vi "Camera_Config_Global_Attributes_2.0.vi"(7 "Camera":T5, 8 "error in (no error)":errorcluster, 10 "Refnum in":T2, 11 "Data":T1={"Camera 1"={"Camera1"="", "Cam 1"=FALSE, "CAM1 Model"=enum."a2A5328-15ucBAS", "Cam1 ID"=0}, "Camera 2"={"Camera2"="", "Cam 2"=FALSE, "CAM2 Model"=enum."a2A5328-15ucBAS", "Cam2 ID"=0}, "Image"={"Camera1_Img"=refnum, "Camera2_Img"=refnum, "Img1_Orig_Disp"=refnum, "Img2_Orig_Disp"=refnum, "Img1_Orig_RGB"=refnum, "Img2_Orig_RGB"=refnum, "Blue_Plane_Extract"=refnum, "Subtracted_Plane"=refnum, "Img1_Binary"=refnum, "Img2_Binary"=refnum, "Crop_Mask"=refnum, "Img1_Save"=refnum, "Img2_Save"=refnum, "Img1_Cali_Full"=refnum, "Img2_Cali_Full"=refnum, "Img1_Cali_Detect"=refnum, "Img2_Cali_Detect"=refnum}, "Ques"={"Cam 1 queue"=refnum, "Cam 2 queue"=refnum, "Cam 1 - save queue"=refnum, "Cam 2 - save queue"=refnum, "Image Process Queue Size"=500, "Image Save Queue Size"=500, "Overload threshold"=500, "Max large object threshold"=0}, "Arduino SRS"={"Pinch-valve"="", "Actuator"=FALSE, "Open(T)/Close(F)"=FALSE, "Arduino Uno"=""}, "Pump"={"Port"="", "Connection"=FALSE, "Flush Size"=0, "Command"="", "Pump Size"=enum."None", "Pump"=""}, "Camera settings"={"Detection settings"={"Sample size threshold"=500, "Detection Region %"=30.0, "Timeout Sample"=200}, "Lens/camera settings"={"Aperture"=enum."Item 0", "Legacy Cam Attributes"=FALSE, "Max Framerate"=100, "Exposure Time"=1000.0, "Framerate"=15}, "Crop settings"={"Cam1"={"Rectangle 1"={"Left"=0, "Top"=0, "Right"=0, "Bottom"=0, "Rotation"=0.0}, "Camera Orientation 1"="", "Pixel to mm 1"=0.0}, "Cam2"={"Rectangle 2"={"Left"=0, "Top"=0, "Right"=0, "Bottom"=0, "Rotation"=0.0}, "Camera Orientation 2"="", "Pixel to mm 2"=0.0}}}, "Arduino ISS"={"Mega F3"="", "Phase3"=FALSE, "Barcode"="", "Sorting sys."=FALSE, "Initial size"=0.0, "Size Interval"=0.0, "Mun. of containers"=0.0, "Container nr."=0.0, "Arduino Mega"=""}, "Img_Capt"=FALSE, "Empty_Refill"=FALSE, "I don't think is in use"={"Light intensity"=100}, "Extended setup"={"Location"="Station", "Latitude"="Station", "Longitude"="Station", "Determiner"="Station", "Sex"="Station", "Station"="", "Collection date"=""}, "Main interface"={"Sample Name"="Test Sample", "Operator"="JFR", "Species Name"="", "Other Notes"=""}, "Tap1"=0, "SystemVersion"=0, "System Serial"="", "Exit"=FALSE, "Kuvette Full"=FALSE, "Core JKI"={"Current VI Reference"=refnum, "Close Panel on Exit?"=FALSE}, "Calibration"={"Calibration 1"=path "C:/Users/au540322/Desktop/IHS_Project/images/Debris/Debris_0/Debris_0_2019_06_01-23-32-49-686.PNG", "Calibration 2"=path "C:/Users/au540322/Desktop/IHS_Project/images/Debris/Debris_0/Debris_0_2019_06_01-23-32-49-686.PNG", "Detect 1"=path "C:/Users/au540322/Desktop/IHS_Project/images/Debris/Debris_0/Debris_0_2019_06_01-23-32-49-686.PNG", "Detect 2"=path "C:/Users/au540322/Desktop/IHS_Project/images/Debris/Debris_0/Debris_0_2019_06_01-23-32-49-686.PNG"}, "Flush Insect"=FALSE, "Auto Flush"=FALSE} {"SystemVersion" items=["Standard", "XL"]; "Tap1" items=["Session Data", "Extended Setup", "Buffer", "Camera", "Dispenser", "Stats", "Connections"]; "I don't think is in use"."Light intensity" scale=0.0..100.0; "Camera settings"."Crop settings"."Cam2"."Rectangle 2"."Rotation" format="%.2f"; "Camera settings"."Crop settings"."Cam2"."Rectangle 2"."Left" scale=0.0..1024.0; "Camera settings"."Crop settings"."Cam2"."Rectangle 2"."Right" scale=0.0..1024.0; "Camera settings"."Crop settings"."Cam1"."Rectangle 1"."Rotation" format="%.2f"; "Camera settings"."Crop settings"."Cam1"."Rectangle 1"."Left" scale=0.0..1024.0; "Camera settings"."Crop settings"."Cam1"."Rectangle 1"."Right" scale=0.0..1024.0; "Camera settings"."Lens/camera settings"."Framerate" min=1; "Camera settings"."Lens/camera settings"."Max Framerate" min=1; "Camera settings"."Detection settings"."Sample size threshold" min=1; "Pump"."Flush Size" min=0 max=6000 step=100; "Ques"."Overload threshold" min=1; "Ques"."Image Save Queue Size" min=1; "Ques"."Image Process Queue Size" min=1}) -> (0 "error out":errorcluster, 2 "Refnum out":T2, 3 "Data Out":T1={"Camera 1"={"Camera1"="", "Cam 1"=FALSE, "CAM1 Model"=enum."a2A5328-15ucBAS", "Cam1 ID"=0}, "Camera 2"={"Camera2"="", "Cam 2"=FALSE, "CAM2 Model"=enum."a2A5328-15ucBAS", "Cam2 ID"=0}, "Image"={"Camera1_Img"=refnum, "Camera2_Img"=refnum, "Img1_Orig_Disp"=refnum, "Img2_Orig_Disp"=refnum, "Img1_Orig_RGB"=refnum, "Img2_Orig_RGB"=refnum, "Blue_Plane_Extract"=refnum, "Subtracted_Plane"=refnum, "Img1_Binary"=refnum, "Img2_Binary"=refnum, "Crop_Mask"=refnum, "Img1_Save"=refnum, "Img2_Save"=refnum, "Img1_Cali_Full"=refnum, "Img2_Cali_Full"=refnum, "Img1_Cali_Detect"=refnum, "Img2_Cali_Detect"=refnum}, "Ques"={"Cam 1 queue"=refnum, "Cam 2 queue"=refnum, "Cam 1 - save queue"=refnum, "Cam 2 - save queue"=refnum, "Image Process Queue Size"=500, "Image Save Queue Size"=500, "Overload threshold"=500, "Max large object threshold"=0}, "Arduino SRS"={"Pinch-valve"="", "Actuator"=FALSE, "Open(T)/Close(F)"=FALSE, "Arduino Uno"=""}, "Pump"={"Port"="", "Connection"=FALSE, "Flush Size"=0, "Command"="", "Pump Size"=enum."None", "Pump"=""}, "Camera settings"={"Detection settings"={"Sample size threshold"=500, "Detection Region %"=30.0, "Timeout Sample"=200}, "Lens/camera settings"={"Aperture"=enum."Item 0", "Legacy Cam Attributes"=FALSE, "Max Framerate"=100, "Exposure Time"=1000.0, "Framerate"=15}, "Crop settings"={"Cam1"={"Rectangle 1"={"Left"=0, "Top"=0, "Right"=0, "Bottom"=0, "Rotation"=0.0}, "Camera Orientation 1"="", "Pixel to mm 1"=0.0}, "Cam2"={"Rectangle 2"={"Left"=0, "Top"=0, "Right"=0, "Bottom"=0, "Rotation"=0.0}, "Camera Orientation 2"="", "Pixel to mm 2"=0.0}}}, "Arduino ISS"={"Mega F3"="", "Phase3"=FALSE, "Barcode"="", "Sorting sys."=FALSE, "Initial size"=0.0, "Size Interval"=0.0, "Mun. of containers"=0.0, "Container nr."=0.0, "Arduino Mega"=""}, "Img_Capt"=FALSE, "Empty_Refill"=FALSE, "I don't think is in use"={"Light intensity"=100}, "Extended setup"={"Location"="Station", "Latitude"="Station", "Longitude"="Station", "Determiner"="Station", "Sex"="Station", "Station"="", "Collection date"=""}, "Main interface"={"Sample Name"="Test Sample", "Operator"="JFR", "Species Name"="", "Other Notes"=""}, "Tap1"=0, "SystemVersion"=0, "System Serial"="", "Exit"=FALSE, "Kuvette Full"=FALSE, "Core JKI"={"Current VI Reference"=refnum, "Close Panel on Exit?"=FALSE}, "Calibration"={"Calibration 1"=path "C:/Users/au540322/Desktop/IHS_Project/images/Debris/Debris_0/Debris_0_2019_06_01-23-32-49-686.PNG", "Calibration 2"=path "C:/Users/au540322/Desktop/IHS_Project/images/Debris/Debris_0/Debris_0_2019_06_01-23-32-49-686.PNG", "Detect 1"=path "C:/Users/au540322/Desktop/IHS_Project/images/Debris/Debris_0/Debris_0_2019_06_01-23-32-49-686.PNG", "Detect 2"=path "C:/Users/au540322/Desktop/IHS_Project/images/Debris/Debris_0/Debris_0_2019_06_01-23-32-49-686.PNG"}, "Flush Insect"=FALSE, "Auto Flush"=FALSE} {"SystemVersion" items=["Standard", "XL"]; "Tap1" items=["Session Data", "Extended Setup", "Buffer", "Camera", "Dispenser", "Stats", "Connections"]; "I don't think is in use"."Light intensity" scale=0.0..100.0; "Camera settings"."Crop settings"."Cam2"."Rectangle 2"."Rotation" format="%.2f"; "Camera settings"."Crop settings"."Cam2"."Rectangle 2"."Left" scale=0.0..1024.0; "Camera settings"."Crop settings"."Cam2"."Rectangle 2"."Right" scale=0.0..1024.0; "Camera settings"."Crop settings"."Cam1"."Rectangle 1"."Rotation" format="%.2f"; "Camera settings"."Crop settings"."Cam1"."Rectangle 1"."Left" scale=0.0..1024.0; "Camera settings"."Crop settings"."Cam1"."Rectangle 1"."Right" scale=0.0..1024.0; "Camera settings"."Lens/camera settings"."Framerate" min=1; "Camera settings"."Lens/camera settings"."Max Framerate" min=1; "Camera settings"."Detection settings"."Sample size threshold" min=1; "Pump"."Flush Size" min=0 max=6000 step=100; "Ques"."Overload threshold" min=1; "Ques"."Image Save Queue Size" min=1; "Ques"."Image Process Queue Size" min=1})   [LabVIEW 2024]
uses:
  <vilib>/userDefined/High Color/IMAQdx.ctl
  Camera_ID.ctl
  controls/Data_JKI.ctl
  <vilib>/vision/Image Controls.llb/IMAQ Image.ctl
  <resource>/objmgr/imaqdx.rc
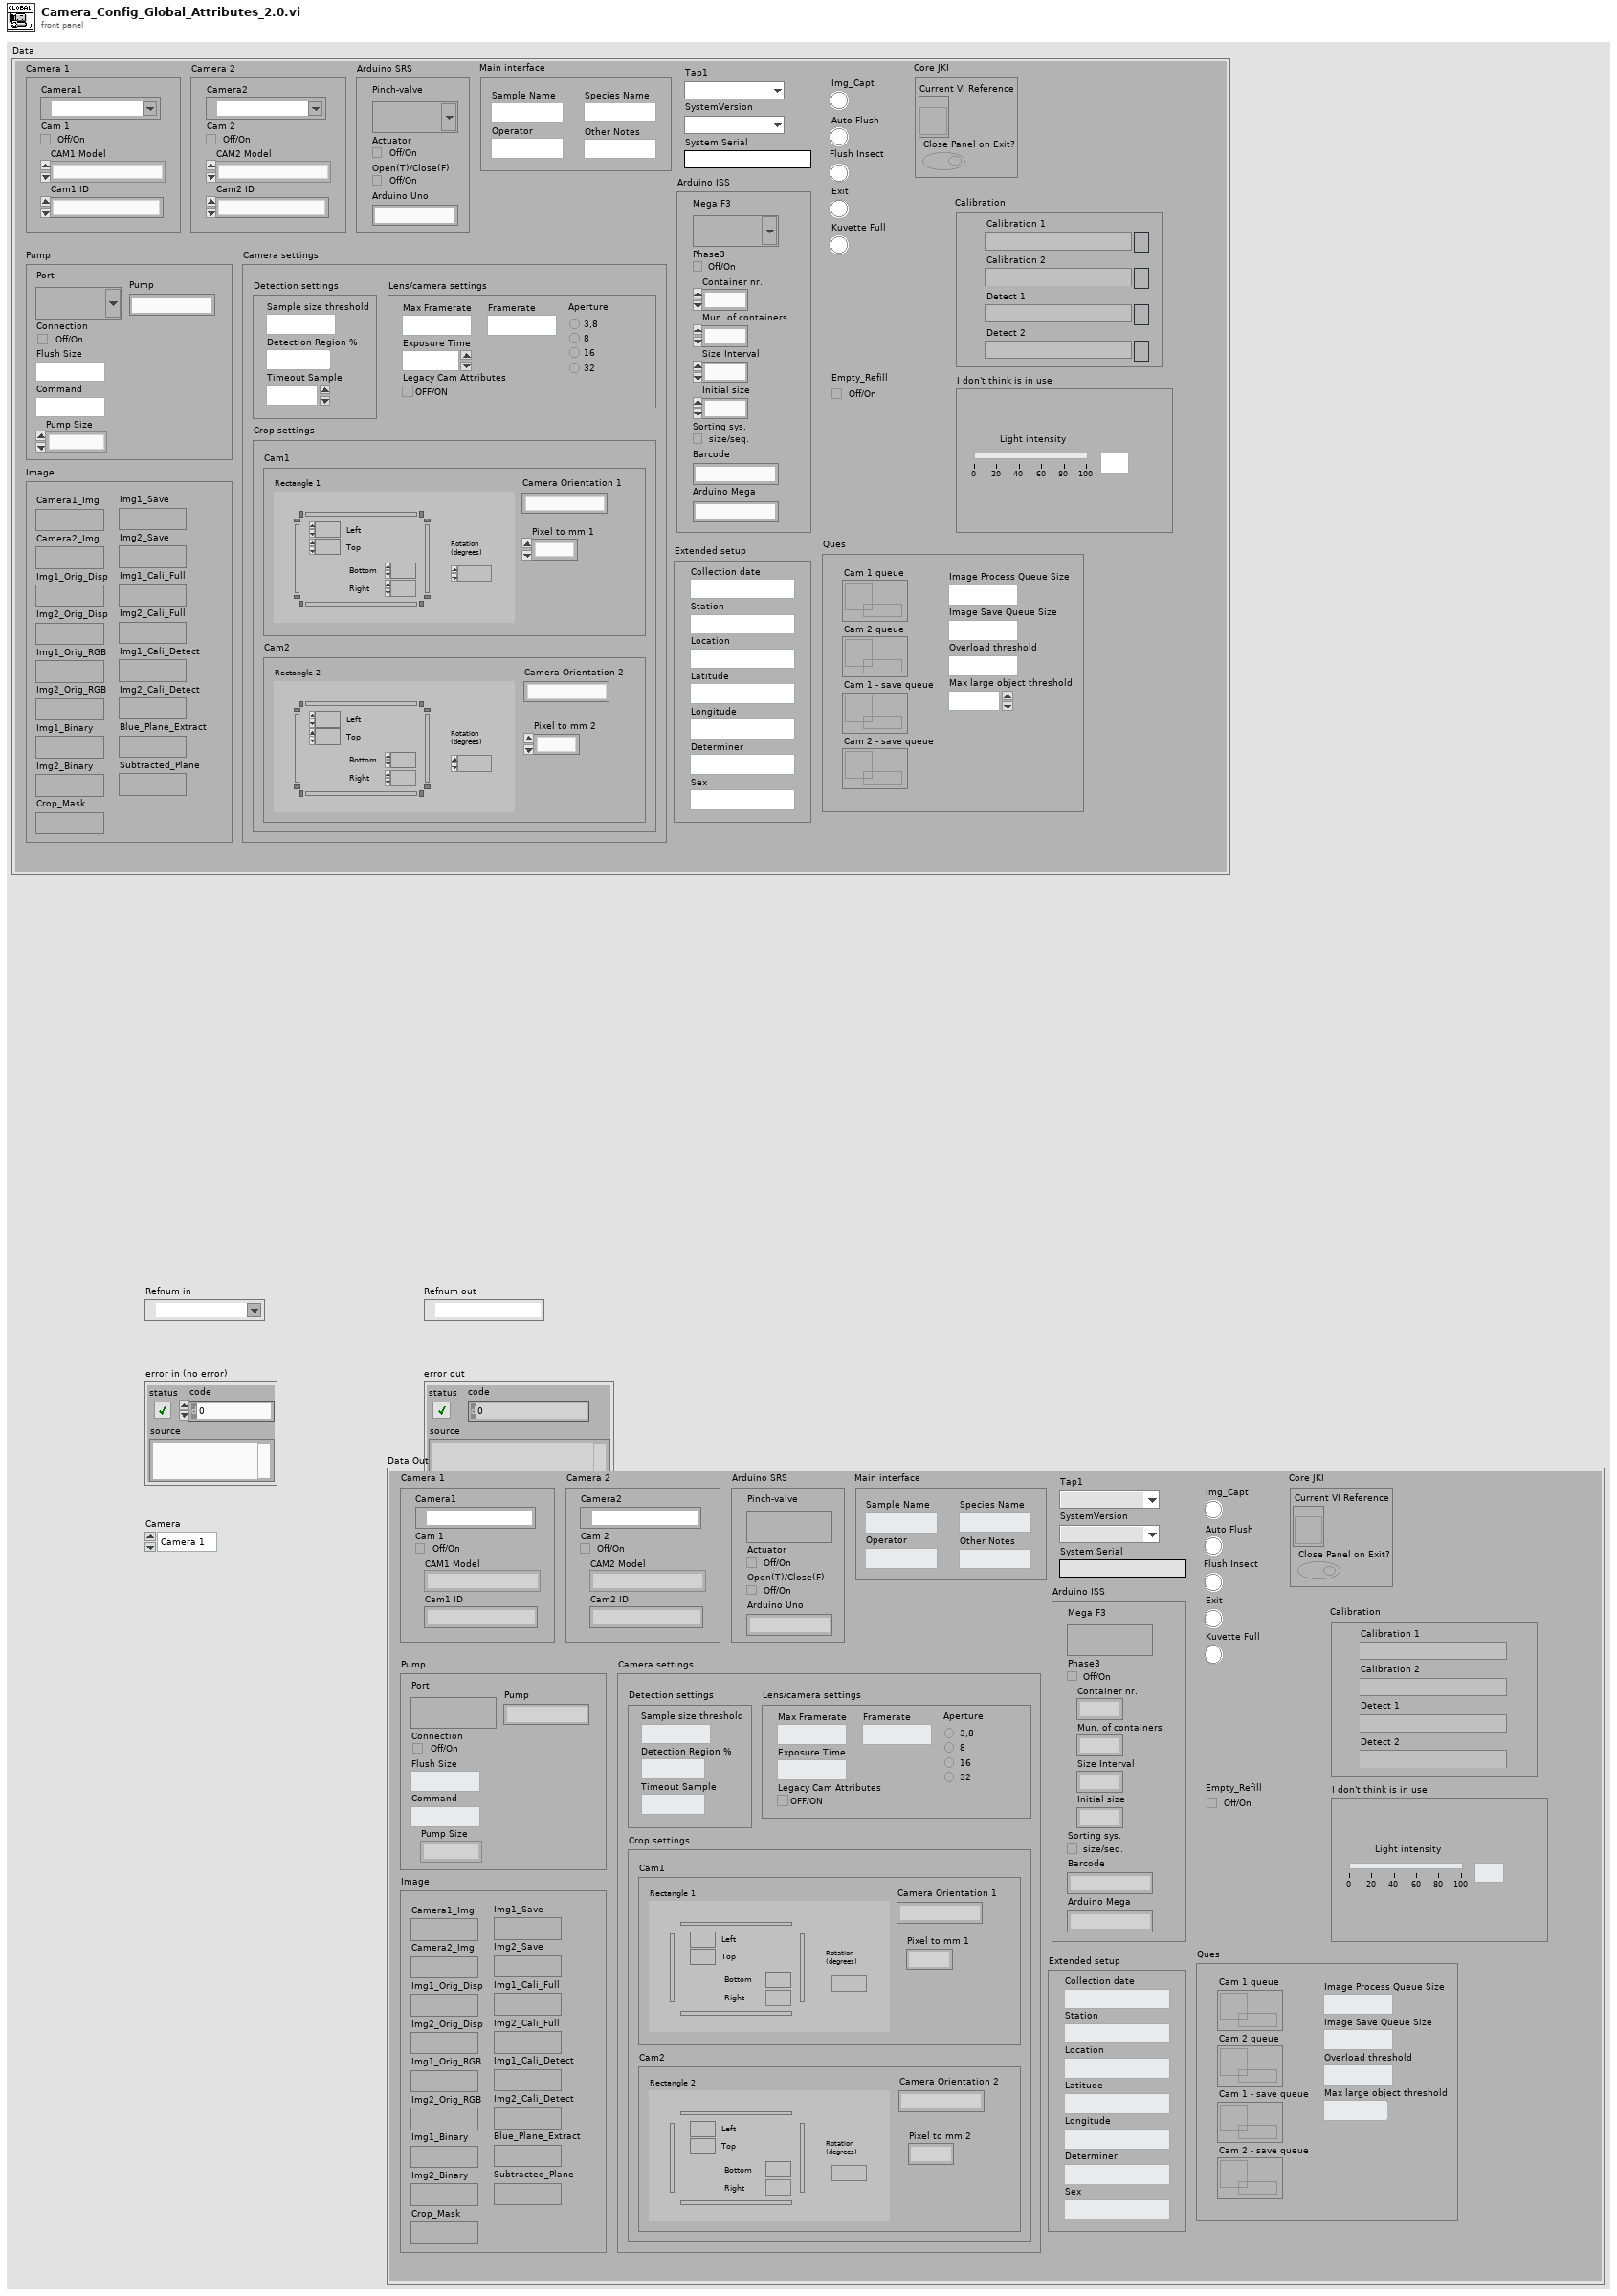
[diagram p1: front panel]
types:
  T1 = typedef "Data_JKI.ctl" = cluster{"Camera 1":cluster{"Camera1":T2, "Cam 1":bool, "CAM1 Model":enum16{"a2A5328-15ucBAS", "acA1920-155uc"}, "Cam1 ID":i32}, "Camera 2":cluster{"Camera2":T2, "Cam 2":bool, "CAM2 Model":enum16{"a2A5328-15ucBAS", "acA1920-155uc"}, "Cam2 ID":i32}, "Image":cluster{"Camera1_Img":T3, "Camera2_Img":T3, "Img1_Orig_Disp":T3, "Img2_Orig_Disp":T3, "Img1_Orig_RGB":T3, "Img2_Orig_RGB":T3, "Blue_Plane_Extract":T3, "Subtracted_Plane":T3, "Img1_Binary":T3, "Img2_Binary":T3, "Crop_Mask":T3, "Img1_Save":T3, "Img2_Save":T3, "Img1_Cali_Full":T3, "Img2_Cali_Full":T3, "Img1_Cali_Detect":T3, "Img2_Cali_Detect":T3}, "Ques":cluster{"Cam 1 queue":refnum<queue>, "Cam 2 queue":refnum<queue>, "Cam 1 - save queue":refnum<queue>, "Cam 2 - save queue":refnum<queue>, "Image Process Queue Size":i32, "Image Save Queue Size":i32, "Overload threshold":i32, "Max large object threshold":i32}, "Arduino SRS":cluster{"Pinch-valve":refnum<visa-resource-name>, "Actuator":bool, "Open(T)/Close(F)":bool, "Arduino Uno":string}, "Pump":cluster{"Port":refnum<visa-resource-name>, "Connection":bool, "Flush Size":i32, "Command":string, "Pump Size":enum16{"None", "Small", "Large"}, "Pump":string}, "Camera settings":cluster{"Detection settings":cluster{"Sample size threshold":i32, "Detection Region %":dbl, "Timeout Sample":i32}, "Lens/camera settings":cluster{"Aperture":enum32{"Item 0", "Item 1", "Item 2", "Item 3"}, "Legacy Cam Attributes":bool, "Max Framerate":i32, "Exposure Time":dbl, "Framerate":i32}, "Crop settings":cluster{"Cam1":cluster{"Rectangle 1":T4, "Camera Orientation 1":string, "Pixel to mm 1":dbl}, "Cam2":cluster{"Rectangle 2":T4, "Camera Orientation 2":string, "Pixel to mm 2":dbl}}}, "Arduino ISS":cluster{"Mega F3":refnum<visa-resource-name>, "Phase3":bool, "Barcode":string, "Sorting sys.":bool, "Initial size":dbl, "Size Interval":dbl, "Mun. of containers":dbl, "Container nr.":dbl, "Arduino Mega":string}, "Img_Capt":bool, "Empty_Refill":bool, "I don't think is in use":cluster{"Light intensity":i32}, "Extended setup":cluster{"Location":string, "Latitude":string, "Longitude":string, "Determiner":string, "Sex":string, "Station":string, "Collection date":string}, "Main interface":cluster{"Sample Name":string, "Operator":string, "Species Name":string, "Other Notes":string}, "Tap1":u16, "SystemVersion":u16, "System Serial":string, "Exit":bool, "Kuvette Full":bool, "Core JKI":cluster{"Current VI Reference":refnum<vi>, "Close Panel on Exit?":bool}, "Calibration":cluster{"Calibration 1":path, "Calibration 2":path, "Detect 1":path, "Detect 2":path}, "Flush Insect":bool, "Auto Flush":bool}
  T2 = typedef "IMAQdx.ctl" = refnum<k21>
  T3 = typedef "IMAQ Image.ctl" = refnum<image>
  T4 = typedef "IMAQ Rectangle" = cluster{"Left":i32, "Top":i32, "Right":i32, "Bottom":i32, "Rotation":dbl}
  T5 = typedef "Camera_ID.ctl" = enum16{"Camera 1", "Camera 2"}
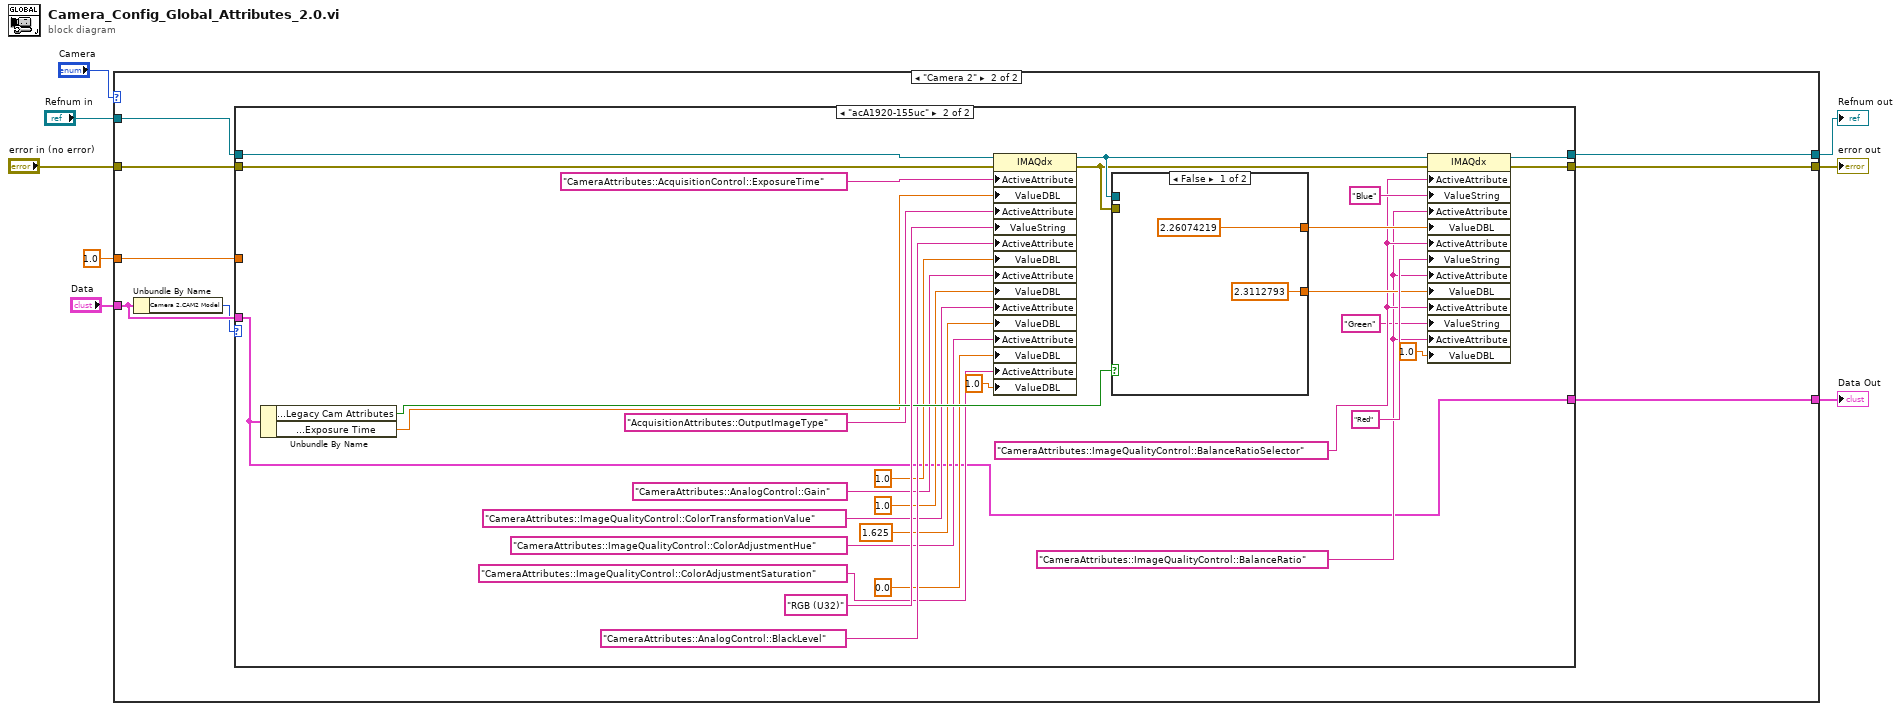
[diagram p0: block diagram]
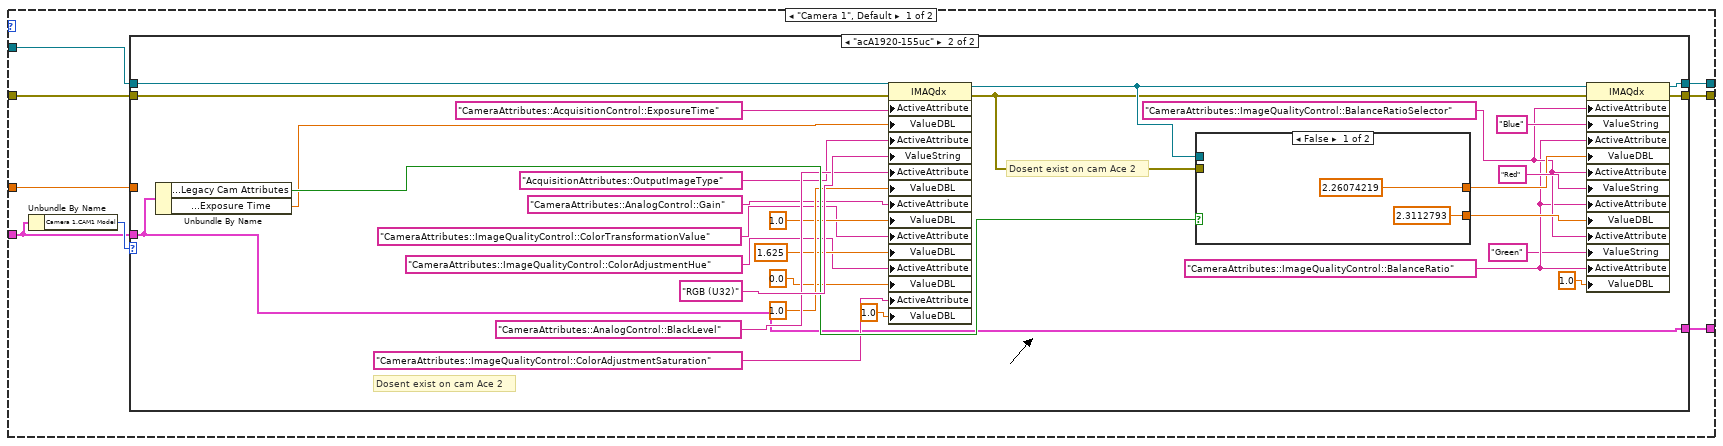
[diagram p2: hidden frame]
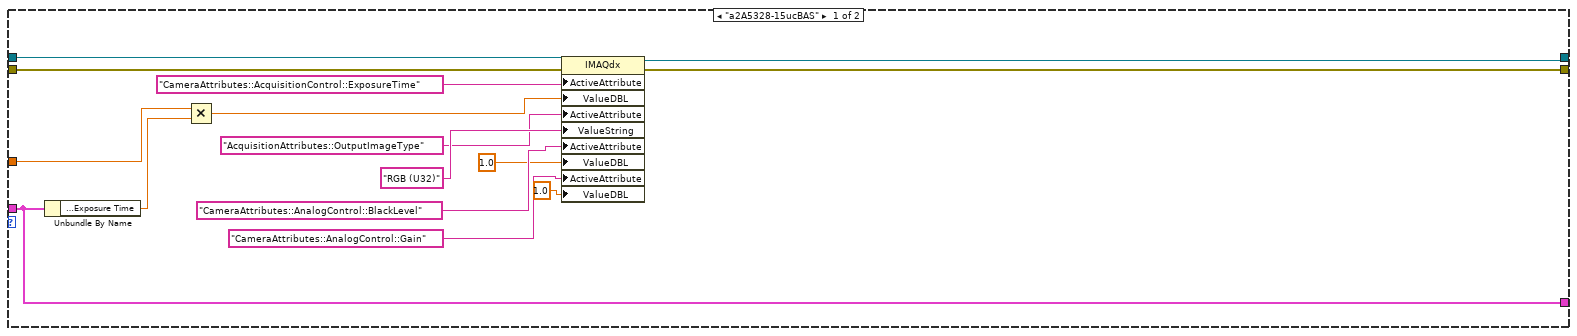
[diagram p3: hidden frame]
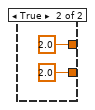
[diagram p4: hidden frame]
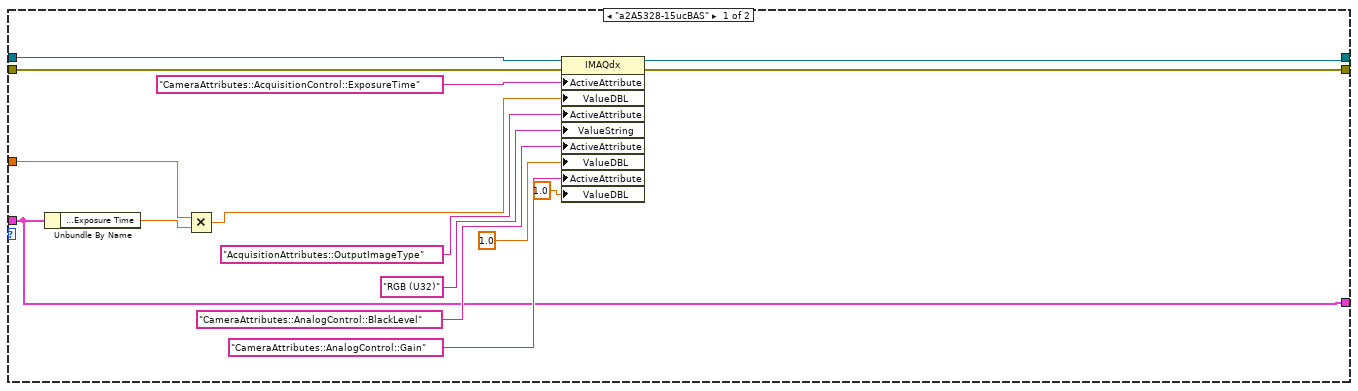
[diagram p5: hidden frame]
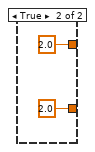
[diagram p6: hidden frame]
diagram:
  n1 = case shown="\"Camera 2\"" "Camera" {
    tunnel: "Data" -> [w13 w73]
    tunnel: "error in (no error)" -> [w14 w72]
    tunnel: [w15 w71] -> w7
    tunnel: "Refnum in" -> [w10 w69]
    tunnel: [w12 w68] -> w4
    tunnel: [w11 w67] -> w3
    tunnel: 1.0 ("x") -> [w9 w66]
    frame "Camera 1", Default {
      n2 = Unbundle By Name(w13) -> ("Camera 1.CAM1 Model"=w16:enum16{"a2A5328-15ucBAS", "acA1920-155uc"})
      n3 = case shown="\"acA1920-155uc\"" w16 {
        tunnel: w13 -> [w27 w34]
        tunnel: w14 -> [w31 w37]
        tunnel: [w29 w36] -> w15
        tunnel: [w27 w34] -> w12
        tunnel: [w28 w35] -> w11
        tunnel: w10 -> [w30 w33]
        tunnel: w9 -> [w19 _]
        frame "a2A5328-15ucBAS" {
          n4 = Unbundle By Name(w27) -> ("Camera settings.Lens/camera settings.Exposure Time"=w18:dbl)
          n5 = Multiply(x=w19, y=w18) -> (x*y=w17:dbl)
          n6 = property class="IMAQdx"(reference=w30, error in=w31, "ActiveAttribute"="CameraAttributes::AcquisitionControl::ExposureTime", "ValueDBL"=w17, "ActiveAttribute"="AcquisitionAttributes::OutputImageType", "ValueString"="RGB (U32)", "ActiveAttribute"="CameraAttributes::AnalogControl::BlackLevel", "ValueDBL"=1.0, "ActiveAttribute"="CameraAttributes::AnalogControl::Gain", "ValueDBL"=1.0) -> (reference out=w28:T2, error out=w29:errorcluster)
        }
        frame "acA1920-155uc" {
          w42 = "CameraAttributes::ImageQualityControl::BalanceRatio" ("ActiveAttribute")
          w43 = "CameraAttributes::ImageQualityControl::BalanceRatioSelector" ("ActiveAttribute")
          # "Dosent exist on cam Ace 2"
          # "Dosent exist on cam Ace 2"
          n7 = Unbundle By Name(w34) -> ("Camera settings.Lens/camera settings.Legacy Cam Attributes"=w58:bool, "Camera settings.Lens/camera settings.Exposure Time"=w32:dbl)
          n8 = property class="IMAQdx"(reference=w33, error in=w37, "ActiveAttribute"="CameraAttributes::AcquisitionControl::ExposureTime", "ValueDBL"=w32, "ActiveAttribute"="AcquisitionAttributes::OutputImageType", "ValueString"="RGB (U32)", "ActiveAttribute"="CameraAttributes::AnalogControl::BlackLevel", "ValueDBL"=1.0, "ActiveAttribute"="CameraAttributes::AnalogControl::Gain", "ValueDBL"=1.0, "ActiveAttribute"="CameraAttributes::ImageQualityControl::ColorTransformationValue", "ValueDBL"=1.625, "ActiveAttribute"="CameraAttributes::ImageQualityControl::ColorAdjustmentHue", "ValueDBL"=0.0, "ActiveAttribute"="CameraAttributes::ImageQualityControl::ColorAdjustmentSaturation", "ValueDBL"=1.0) -> (reference out=w60:T2, error out=w59:errorcluster)
          n9 = case shown="False" w58 {
            tunnel: w60 -> [_ _]
            tunnel: w59 -> [_ _]
            tunnel: [2.26074219 ("ValueDBL") 2.0 ("ValueDBL")] -> w55
            tunnel: [2.3112793 ("ValueDBL") 2.0 ("ValueDBL")] -> w54
            frame False {
            }
            frame True {
            }
          }
          n10 = property class="IMAQdx"(reference=w60, error in=w59, "ActiveAttribute"=w43, "ValueString"="Blue", "ActiveAttribute"=w42, "ValueDBL"=w55, "ActiveAttribute"=w43, "ValueString"="Red", "ActiveAttribute"=w42, "ValueDBL"=w54, "ActiveAttribute"=w43, "ValueString"="Green", "ActiveAttribute"=w42, "ValueDBL"=1.0) -> (reference out=w35:T2, error out=w36:errorcluster)
        }
      }
    }
    frame "Camera 2" {
      n11 = Unbundle By Name(w73) -> ("Camera 2.CAM2 Model"=w70:enum16{"a2A5328-15ucBAS", "acA1920-155uc"})
      n12 = case shown="\"acA1920-155uc\"" w70 {
        tunnel: w73 -> [w79 w90]
        tunnel: w72 -> [w81 w94]
        tunnel: [w78 w93] -> w71
        tunnel: w69 -> [w80 w91]
        tunnel: [w79 w90] -> w68
        tunnel: [w77 w92] -> w67
        tunnel: w66 -> [w74 _]
        frame "a2A5328-15ucBAS" {
          n13 = Unbundle By Name(w79) -> ("Camera settings.Lens/camera settings.Exposure Time"=w76:dbl)
          n14 = Multiply(x=w74, y=w76) -> (x*y=w75:dbl)
          n15 = property class="IMAQdx"(reference=w80, error in=w81, "ActiveAttribute"="CameraAttributes::AcquisitionControl::ExposureTime", "ValueDBL"=w75, "ActiveAttribute"="AcquisitionAttributes::OutputImageType", "ValueString"="RGB (U32)", "ActiveAttribute"="CameraAttributes::AnalogControl::BlackLevel", "ValueDBL"=1.0, "ActiveAttribute"="CameraAttributes::AnalogControl::Gain", "ValueDBL"=1.0) -> (reference out=w77:T2, error out=w78:errorcluster)
        }
        frame "acA1920-155uc" {
          w99 = "CameraAttributes::ImageQualityControl::BalanceRatio" ("ActiveAttribute")
          w100 = "CameraAttributes::ImageQualityControl::BalanceRatioSelector" ("ActiveAttribute")
          n16 = Unbundle By Name(w90) -> ("Camera settings.Lens/camera settings.Legacy Cam Attributes"=w115:bool, "Camera settings.Lens/camera settings.Exposure Time"=w89:dbl)
          n17 = property class="IMAQdx"(reference=w91, error in=w94, "ActiveAttribute"="CameraAttributes::AcquisitionControl::ExposureTime", "ValueDBL"=w89, "ActiveAttribute"="AcquisitionAttributes::OutputImageType", "ValueString"="RGB (U32)", "ActiveAttribute"="CameraAttributes::AnalogControl::BlackLevel", "ValueDBL"=1.0, "ActiveAttribute"="CameraAttributes::AnalogControl::Gain", "ValueDBL"=1.0, "ActiveAttribute"="CameraAttributes::ImageQualityControl::ColorTransformationValue", "ValueDBL"=1.625, "ActiveAttribute"="CameraAttributes::ImageQualityControl::ColorAdjustmentHue", "ValueDBL"=0.0, "ActiveAttribute"="CameraAttributes::ImageQualityControl::ColorAdjustmentSaturation", "ValueDBL"=1.0) -> (reference out=w117:T2, error out=w116:errorcluster)
          n18 = case shown="False" w115 {
            tunnel: w117 -> [_ _]
            tunnel: w116 -> [_ _]
            tunnel: [2.26074219 ("ValueDBL") 2.0 ("ValueDBL")] -> w112
            tunnel: [2.3112793 ("ValueDBL") 2.0 ("ValueDBL")] -> w111
            frame False {
            }
            frame True {
            }
          }
          n19 = property class="IMAQdx"(reference=w117, error in=w116, "ActiveAttribute"=w100, "ValueString"="Blue", "ActiveAttribute"=w99, "ValueDBL"=w112, "ActiveAttribute"=w100, "ValueString"="Red", "ActiveAttribute"=w99, "ValueDBL"=w111, "ActiveAttribute"=w100, "ValueString"="Green", "ActiveAttribute"=w99, "ValueDBL"=1.0) -> (reference out=w92:T2, error out=w93:errorcluster)
        }
      }
    }
  }
  "error out" <- w7
  "Refnum out" <- w3
  "Data Out" <- w4
